vi "Set File Properties.vi"(8 "error in (no error)":errorcluster, 11 "Data Logger Module in":refnum<class "Data Logger DBL Module.lvclass">) -> (0 "error out":errorcluster, 3 "Data Logger Module out":refnum<class "Data Logger DBL Module.lvclass">)   [LabVIEW 2020, in "VolatusData.lvlib" / "Data Logger DBL Module.lvclass"]
uses:
  Data Logger DBL Module.lvclass
  C:/dev/lv20CE/relink/lv-volatus/Volatus/Module/Module.lvclass
  Volatus/Module/Module.lvclass/Module.ctl
  Data Logger DBL Module.lvclass/Data Logger DBL Module.ctl
  Volatus/Module/Module.lvclass
  Volatus/VolatusAPI/VolatusAPI.lvclass
  VolatusConfig/VolatusConfig/VolatusConfig.lvclass
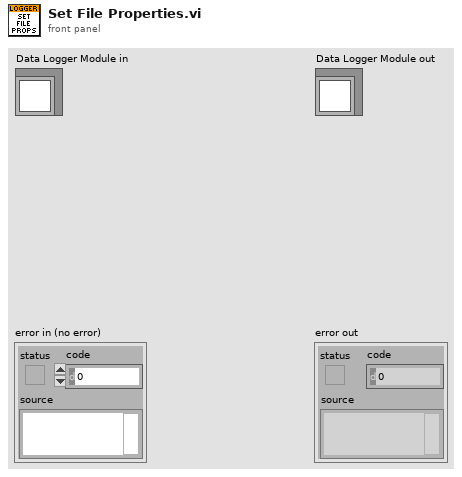
[diagram p1: front panel]
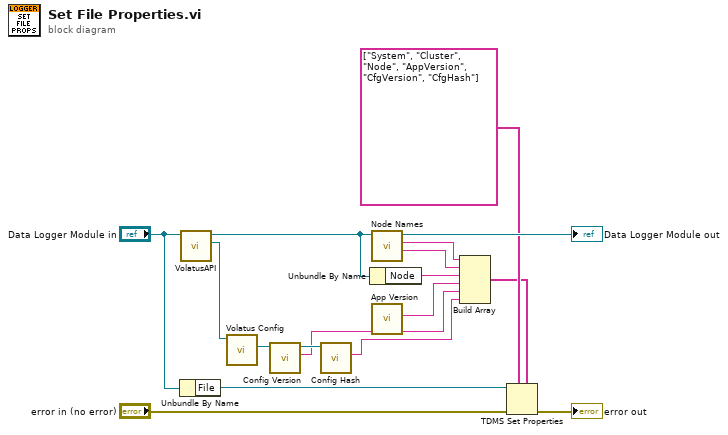
[diagram p0: block diagram]
diagram:
  n1 = Unbundle By Name("Data Logger Module in") -> ("File"=w15:refnum<k34>)
  n2 = call "VolatusAPI.vi"("Module in"="Data Logger Module in") -> ("VolatusAPI"=w7:refnum<class "VolatusAPI.lvclass">, "Module out"=w2:refnum<class "Data Logger DBL Module.lvclass">)  [unwired: 9 in]
  n3 = call "Volatus Config.vi"("VolatusAPI in"=w7) -> ("Volatus Config"=w6:refnum<class "VolatusConfig.lvclass">)  [unwired: 8 in, 2 out]
  n4 = call "Config Version.vi"("VolatusConfig in"=w6) -> ("Config Version"=w4:string, "VolatusConfig out"=w5:refnum<class "VolatusConfig.lvclass">)  [unwired: 8 in, 1 out]
  n5 = call "Config Hash.vi"("VolatusConfig in"=w5) -> ("Config Hash"=w3:string)  [unwired: 8 in, 2 out]
  n6 = Unbundle By Name(w2) -> ("Node"=w1:string)
  n7 = call "Node Names.vi"("Module in"=w2) -> ("Cluster"=w10:string, "System"=w11:string, "Module out"=→"Data Logger Module out":refnum<class "Data Logger DBL Module.lvclass">)  [unwired: 6 in, 2 out]
  n8 = call "App Version.vi"() -> ("App Version"=w8:string)  [unwired: 11 in]
  n9 = Build Array(w11, w10, w1, w8, w4, w3) -> (w9:string[])
  n10 = TDMS Set Properties(5:w9, 7:string[] ["System", "Cluster", "Node", "AppVersion", "CfgVersion", "CfgHash"], 8:"error in (no error)", 11:w15) -> (0:→"error out":errorcluster)  [unwired: 2 in, 3 out]
